vi "globalGenerador6_HMI.vi"() -> ()   [LabVIEW 2018]
uses:
  Controls/Cluster_HMI_VIFP - 2.ctl
  <vilib>/RAFA Solutions/Harmony UI Controls Kit/Numeric/Horizontal Progress Bar.ctl
  <vilib>/RAFA Solutions/Harmony UI Controls Kit/Numeric/Numeric Indicator.ctl
  <vilib>/RAFA Solutions/Harmony UI Controls Kit/Flat UI Design.lvlib
panel:
  out "Generador6_HMI":T1 {"I1" scale=0.0..1200.0; "L1" scale=0.0..600.0; "Factor de Potencia" format="%#.1f"; "Potencia Total [kW]" format="%#.1f"; "Frecuencia [Hz]" format="%#.1f"; "I3" scale=0.0..1200.0; "I2" scale=0.0..1200.0; "L3" scale=0.0..600.0; "L2" scale=0.0..600.0}
  # "VOLTAJES [Vrms]"
  # "CORRIENTES [Arms]"
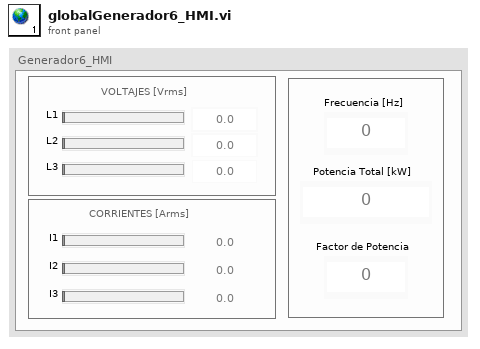
[diagram p1: front panel]
types:
  T1 = typedef "Cluster_HMI_VIFP - 2.ctl" = cluster{"L2":T2, "L3":T2, "I2":T2, "I3":T2, "Frecuencia [Hz]":T3, "Potencia Total [kW]":T3, "Factor de Potencia":T3, "L1":T2, "I1":T2}
  T2 = typedef "Flat UI Design.lvlib/Horizontal Progress Bar.ctl" = sgl
  T3 = typedef "Flat UI Design.lvlib/Numeric Indicator.ctl" = sgl
diagram:
